vi "Add Points to Series_DBL-DBL[].vi"(6 "YValuesPerPoint":i32=1, 8 "error in (no error)":errorcluster, 9 "Data":cluster{"X":dbl, "Y":dbl[]}[](array[cluster])=[{"X"=0.0, "Y"=[]}, {"X"=0.0, "Y"=[]}, {"X"=0.0, "Y"=[]}, {"X"=0.0, "Y"=[]}, {"X"=0.0, "Y"=[]}, {"X"=0.0, "Y"=[]}, {"X"=0.0, "Y"=[]}, {"X"=0.0, "Y"=[]}], 10 ".NET MSChart Series":refnum<k24>) -> (0 "error out":errorcluster)   [LabVIEW 2015, in "Graph Extensions MSChart.lvlib"]
uses:
  Graph Extensions MSChart.lvlib
  System.Windows.Forms.DataVisualization
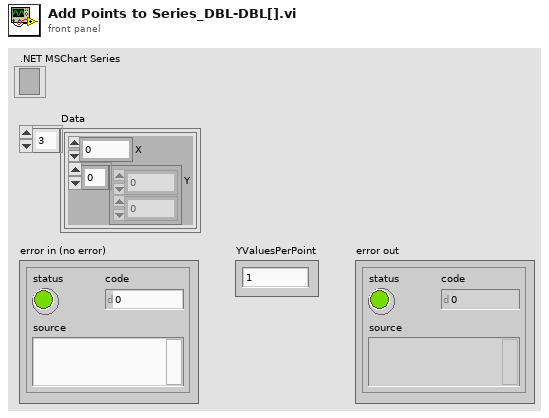
[diagram p1: front panel]
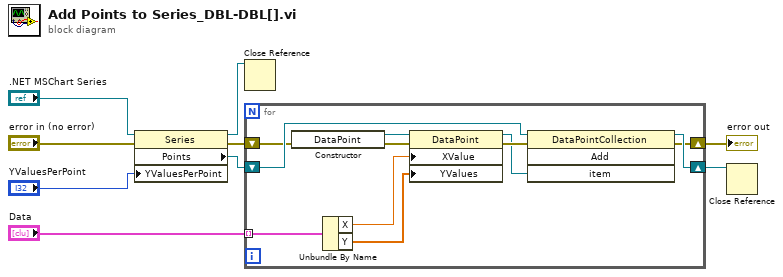
[diagram p0: block diagram]
diagram:
  n1 = property class="Series"(reference=".NET MSChart Series", error in="error in (no error)", "YValuesPerPoint"="YValuesPerPoint") -> (reference out=w6:refnum<k24>, error out=w4:errorcluster, "Points"=w5:refnum<k24>)
  n2 = Close Reference(reference=w6) -> ()  [unwired: 1 in, 1 out]
  n3 = for {
    shift-right: [w19] -> w2
    shift-left: w5 -> [w20]
    shift-right: [w18] -> w1
    shift-left: w4 -> [w14]
    tunnel: "Data" -> [w16] mode=indexing
    n4 = constructor class="DataPoint"(error in=w14) -> (reference out=w17:refnum<k24>, error out=w15:errorcluster)  [unwired: 2 in, 1 out]
    n5 = Unbundle By Name(w16) -> ("X"=w12:dbl, "Y"=w10:dbl[])
    n6 = property class="DataPoint"(reference=w17, error in=w15, "XValue"=w12, "YValues"=w10) -> (reference out=w11:refnum<k24>, error out=w13:errorcluster)
    n7 = invoke class="DataPointCollection" method="Add"(reference=w20, error in=w13, "item"=w11) -> (reference out=w19:refnum<k24>, error out=w18:errorcluster)  [unwired: 1 in, 2 out]
  }
  "error out" <- w1
  n8 = Close Reference(reference=w2) -> ()  [unwired: 1 in, 1 out]
